vi "Main.vi"   [LabVIEW 2019, in "ModuleC.lvlib"]
uses:
  ModuleC.lvlib
  Communication/ACComm/Message5/Message5.lvclass
  Utilities/ArrayUtilities/ArrayUtilities.lvlib
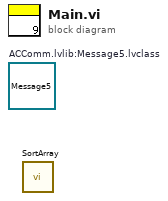
[diagram p0: block diagram]
diagram:
  (unwired) refnum<class "Message5.lvclass"> refnum  # ACComm.lvlib:Message5.lvclass
  n1 = call "SortArray.vi"() -> ()  [unwired: 11 in, 1 out]
